vi "Update_1layer_Wx_FPGA.vi"(1 "Learning rate":fxp<+/-,32,8>, 2 "1layer_Out_hx":fxp<+/-,32,8>, 3 "Array_Weights_hx":fxp<+/-,32,8>[](array[numeric]), 4 "Array_Inputs":fxp<+/-,32,8>[](array[numeric]), 7 "Error OutX":fxp<+/-,32,8>) -> (0 "Array_Weights_hx_updated":fxp<+/-,32,8>[](array[numeric]))   [LabVIEW 2016]
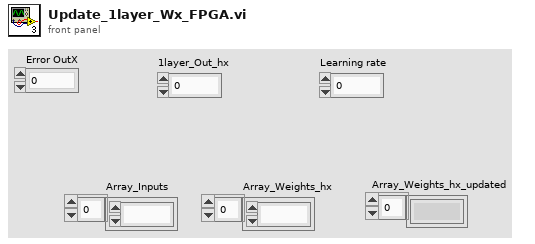
[diagram p1: front panel]
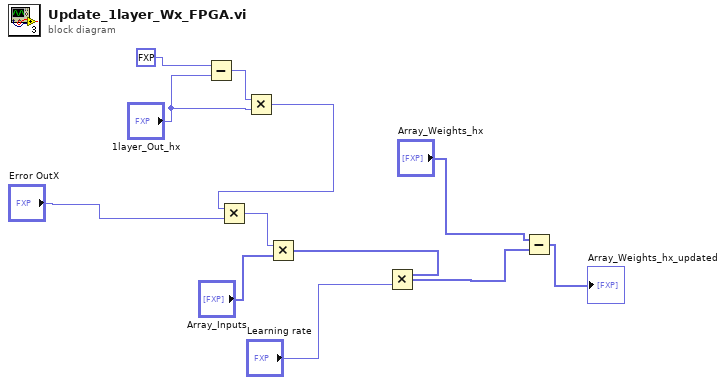
[diagram p0: block diagram]
diagram:
  n1 = Subtract(x=fxp<+,32,8> 1.0, y="1layer_Out_hx") -> (x-y=w10:fxp<+/-,32,8>)
  n2 = Multiply(x=w10, y="1layer_Out_hx") -> (x*y=w12:fxp<+/-,32,8>)
  n3 = Multiply(x=w12, y="Error OutX") -> (x*y=w4:fxp<+/-,32,8>)
  n4 = Multiply(x=w4, y="Array_Inputs") -> (x*y=w6:fxp<+/-,64,16>[])
  n5 = Multiply(x=w6, y="Learning rate") -> (x*y=w8:fxp<+/-,32,8>[])
  n6 = Subtract(x="Array_Weights_hx", y=w8) -> (x-y=→"Array_Weights_hx_updated":fxp<+/-,32,8>[])
